vi "aggregator.vi"(6 "first time":bool=TRUE, 7 "requested size":i32=1, 11 "number":cdb) -> (3 "Array":cdb[](array[numeric]))   [LabVIEW 2018]
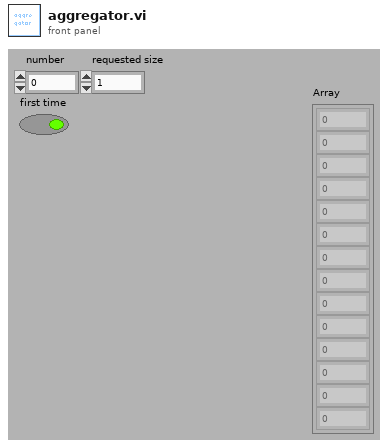
[diagram p1: front panel]
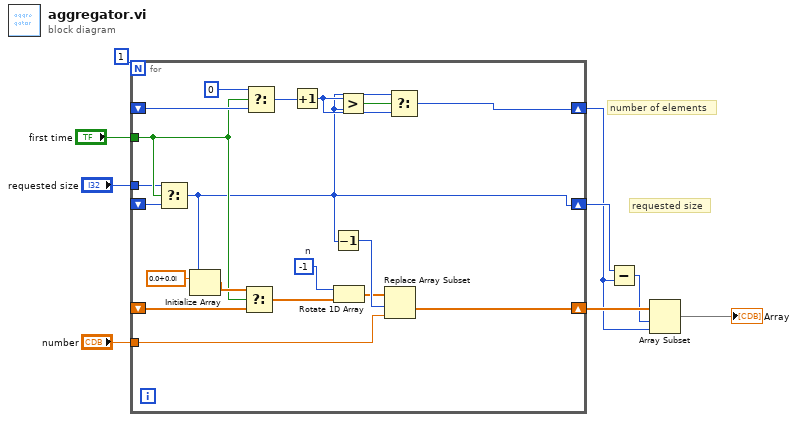
[diagram p0: block diagram]
diagram:
  # "requested size"
  # "number of elements"
  n1 = for {
    N: 1 -> [_]
    tunnel: "first time" -> [w13]
    shift-right: [w25] -> w1
    shift-left: _ -> [w27]
    tunnel: "requested size" -> [w12]
    tunnel: "number" -> [w20]
    shift-right: [w17] -> w5
    shift-left: _ -> [w22]
    shift-right: [w10] -> w3
    shift-left: _ -> [w11]
    w21 = -1  # n
    n2 = Select(t=w12, s=w13, f=w11) -> (s? t:f=w10:i32)
    n3 = Initialize Array(cdb 0.0+0.0i, w10) -> (w14:cdb[])
    n4 = Select(t=w14, s=w13, f=w22) -> (s? t:f=w16:cdb[])
    n5 = Select(t=0, s=w13, f=w27) -> (s? t:f=w24:i32)
    n6 = Increment(x=w24) -> (x+1=w23:i32)
    n7 = Decrement(x=w10) -> (x-1=w19:i32)
    n8 = Rotate 1D Array(1:w16, 2:w21) -> (0:w18:cdb[])
    n9 = Greater?(x=w23, y=w10) -> (0:w26:bool)
    n10 = Replace Array Subset(array=w18, new element=w20, index=w19) -> (w17:cdb[])
    n11 = Select(t=w10, s=w26, f=w23) -> (s? t:f=w25:i32)
  }
  n12 = Subtract(x=w3, y=w1) -> (x-y=w2:i32)
  n13 = Array Subset(array=w5, index=w2, length=w1) -> (→"Array":cdb[])
